vi "createTifFilename.vi"(1 "inputPath":path) -> (0 "tifPath":path)   [LabVIEW 2015]
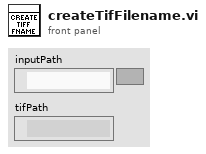
[diagram p1: front panel]
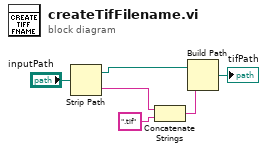
[diagram p0: block diagram]
diagram:
  n1 = Strip Path(path="inputPath") -> (stripped path=w4:path, name=w3:string)
  n2 = Concatenate Strings(w3, ".tif" ("name or relative path")) -> (w2:string)
  n3 = Build Path(base path=w4, name or relative path=w2) -> (appended path=→"tifPath":path)
